vi "Periodic Tasks.vi"(8 "error in":errorcluster) -> ()   [LabVIEW 2012]
doc: "This VI runs in parallel to other tasks. It can contain as many user-defined periodic loops as you need. These can carry out PID or other sorts of timed response."
uses:
  <vilib>/Rock Robotics/SystemInterfaces/Utilities/FPGA_UtilitiesLED Source.ctl
  <vilib>/Rock Robotics/SystemInterfaces/Utilities/FPGA_UtilitiesLED State.ctl
  <vilib>/Rock Robotics/WPI/Solenoid/WPI_SolenoidValue.ctl
  <vilib>/Rock Robotics/WPI/Relay/WPI_RelayValue.ctl
  Robot Global Data.vi
  <vilib>/Rock Robotics/WPI/Solenoid/WPI_SolenoidSetEnum.vi
  <vilib>/Rock Robotics/WPI/Compressor/WPI_CompressorGetSetRefNum.vi
panel:
  out "Pot1 Raw":dbl
  out "Pot1":dbl
  out "PickupError":errorcluster
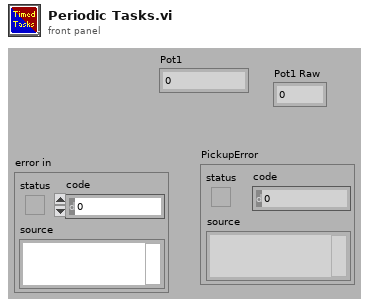
[diagram p1: front panel]
types:
  T1 = typedef "FPGA_UtilitiesLED State.ctl" = enum16{"Off", "On", "Toggle"}
  T2 = typedef "FPGA_UtilitiesLED Source.ctl" = enum16{"User LED", "FPGA LED"}
  T3 = typedef "WPI_SolenoidDevRef.ctl" = cluster{"DevStatus":errorcluster, "Solenoid Module":T4, "Forward Solenoid Channel":T5, "Reverse Solenoid Channel":T5}
  T4 = typedef "FPGA_TypedefSolenoidModule.ctl" = enum16{"Solenoid Module 1", "Solenoid Module 2"}
  T5 = typedef "WPI_SolenoidChannel.ctl" = enum8{"Solenoid 1", "Solenoid 2", "Solenoid 3", "Solenoid 4", "Solenoid 5", "Solenoid 6", "Solenoid 7", "Solenoid 8", "Invalid"}
  T6 = typedef "WPI_RelayDevRef.ctl" = cluster{"DevStatus":errorcluster, "Relay Channel":T7, "Digital Module":T8, "Relay Direction":T9}
  T7 = typedef "FPGA_DIORelayChannel.ctl" = enum8{"Relay 1", "Relay 2", "Relay 3", "Relay 4", "Relay 5", "Relay 6", "Relay 7", "Relay 8", "Invalid"}
  T8 = typedef "FPGA_TypedefDigitalModule.ctl" = enum16{"Digital Module 1", "Digital Module 2"}
  T9 = typedef "WPI_RelayDirection.ctl" = enum16{"Both directions", "Forward only", "Reverse only"}
  T10 = typedef "WPI_MotorControlDeviceRef.ctl" = cluster{"DeviceStatus":errorcluster, "Type":enum16{"PWM", "CAN"}, "PWM":cluster{"Digital Module":T8, "PWM Channel":T11, "DeadBand":T12}, "CAN":cluster{"Device Number":u8, "Control Mode":T13, "Semaphore":T14, "Max Vout":dbl}, "Invert":bool, "TransformRef":T15, "InvTransformRef":T15}
  T11 = typedef "FPGA_DIOPWMChannel.ctl" = enum8{"PWM 1", "PWM 2", "PWM 3", "PWM 4", "PWM 5", "PWM 6", "PWM 7", "PWM 8", "PWM 9", "PWM 10", "Invalid"}
  T12 = typedef "WPI_PWMDeadband.ctl" = cluster{"Name":string, "maxPositivePwm":i32, "minPositivePwm":i32, "centerPwm":i32, "maxNegativePwm":i32, "minNegativePwm":i32, "angularRange":u16}
  T13 = typedef "WPI_CANJaguar_ControlMode.ctl" = enum8{"Percent VBus", "Current", "Speed", "Position", "Voltage"}
  T14 = typedef "Semaphore RefNum" = refnum<k1>
  T15 = typedef "WPI_PWMTransform_ConPane.ctl" = refnum<vi>
  T16 = typedef "WPI_CompressorDevRef.ctl" = cluster{"DevStatus":errorcluster, "DigitalInputDevRef":T17, "RelayDevRef":T6}
  T17 = typedef "WPI_DigitalInputDevRef.ctl" = cluster{"DevStatus":errorcluster, "DIO Channel":T18, "Digital Module":T8}
  T18 = typedef "FPGA_DIOChannel.ctl" = enum8{"DIO 1", "DIO 2", "DIO 3", "DIO 4", "DIO 5", "DIO 6", "DIO 7", "DIO 8", "DIO 9", "DIO 10", "DIO 11", "DIO 12", "DIO 13", "DIO 14", "Invalid"}
  T19 = typedef "WPI_AnalogChannelDevRef.ctl" = cluster{"DevStatus":errorcluster, "Analog Module":T20, "Analog Channel":T21}
  T20 = typedef "FPGA_TypedefAnalogModule.ctl" = enum16{"Analog Module 1", "Analog Module 2"}
  T21 = typedef "FPGA_AIChannel.ctl" = enum8{"AI 1", "AI 2", "AI 3", "AI 4", "AI 5", "AI 6", "AI 7", "AI 8", "Invalid"}
  T22 = enum16{"Reset", "Ready", "Down", "Capture", "Lift", "Swing", "Release"}
  T23 = typedef "WPI_SolenoidValue.ctl" = enum16{"Off", "On", "Forward", "Reverse"}
  T24 = typedef "WPI_RelayValue.ctl" = enum16{"Off", "On", "Forward", "Reverse"}
  T25 = cluster{"PizzaLow":dbl, "PizzaMid":dbl, "PizzaTop":dbl}
  T26 = cluster{"Shoot":bool, "Enable_Targeting":bool, "Shooter":dbl, "LeadScrew":dbl, "Feed":bool, "Pickup":bool, "LiftHooks":bool, "Vision On":bool, "Vision Off":bool, "DownHooks":bool}
  T27 = cluster{"Frisbee_Catch":bool, "Shooter_Ready":bool, "LeadScrewEnd":bool}
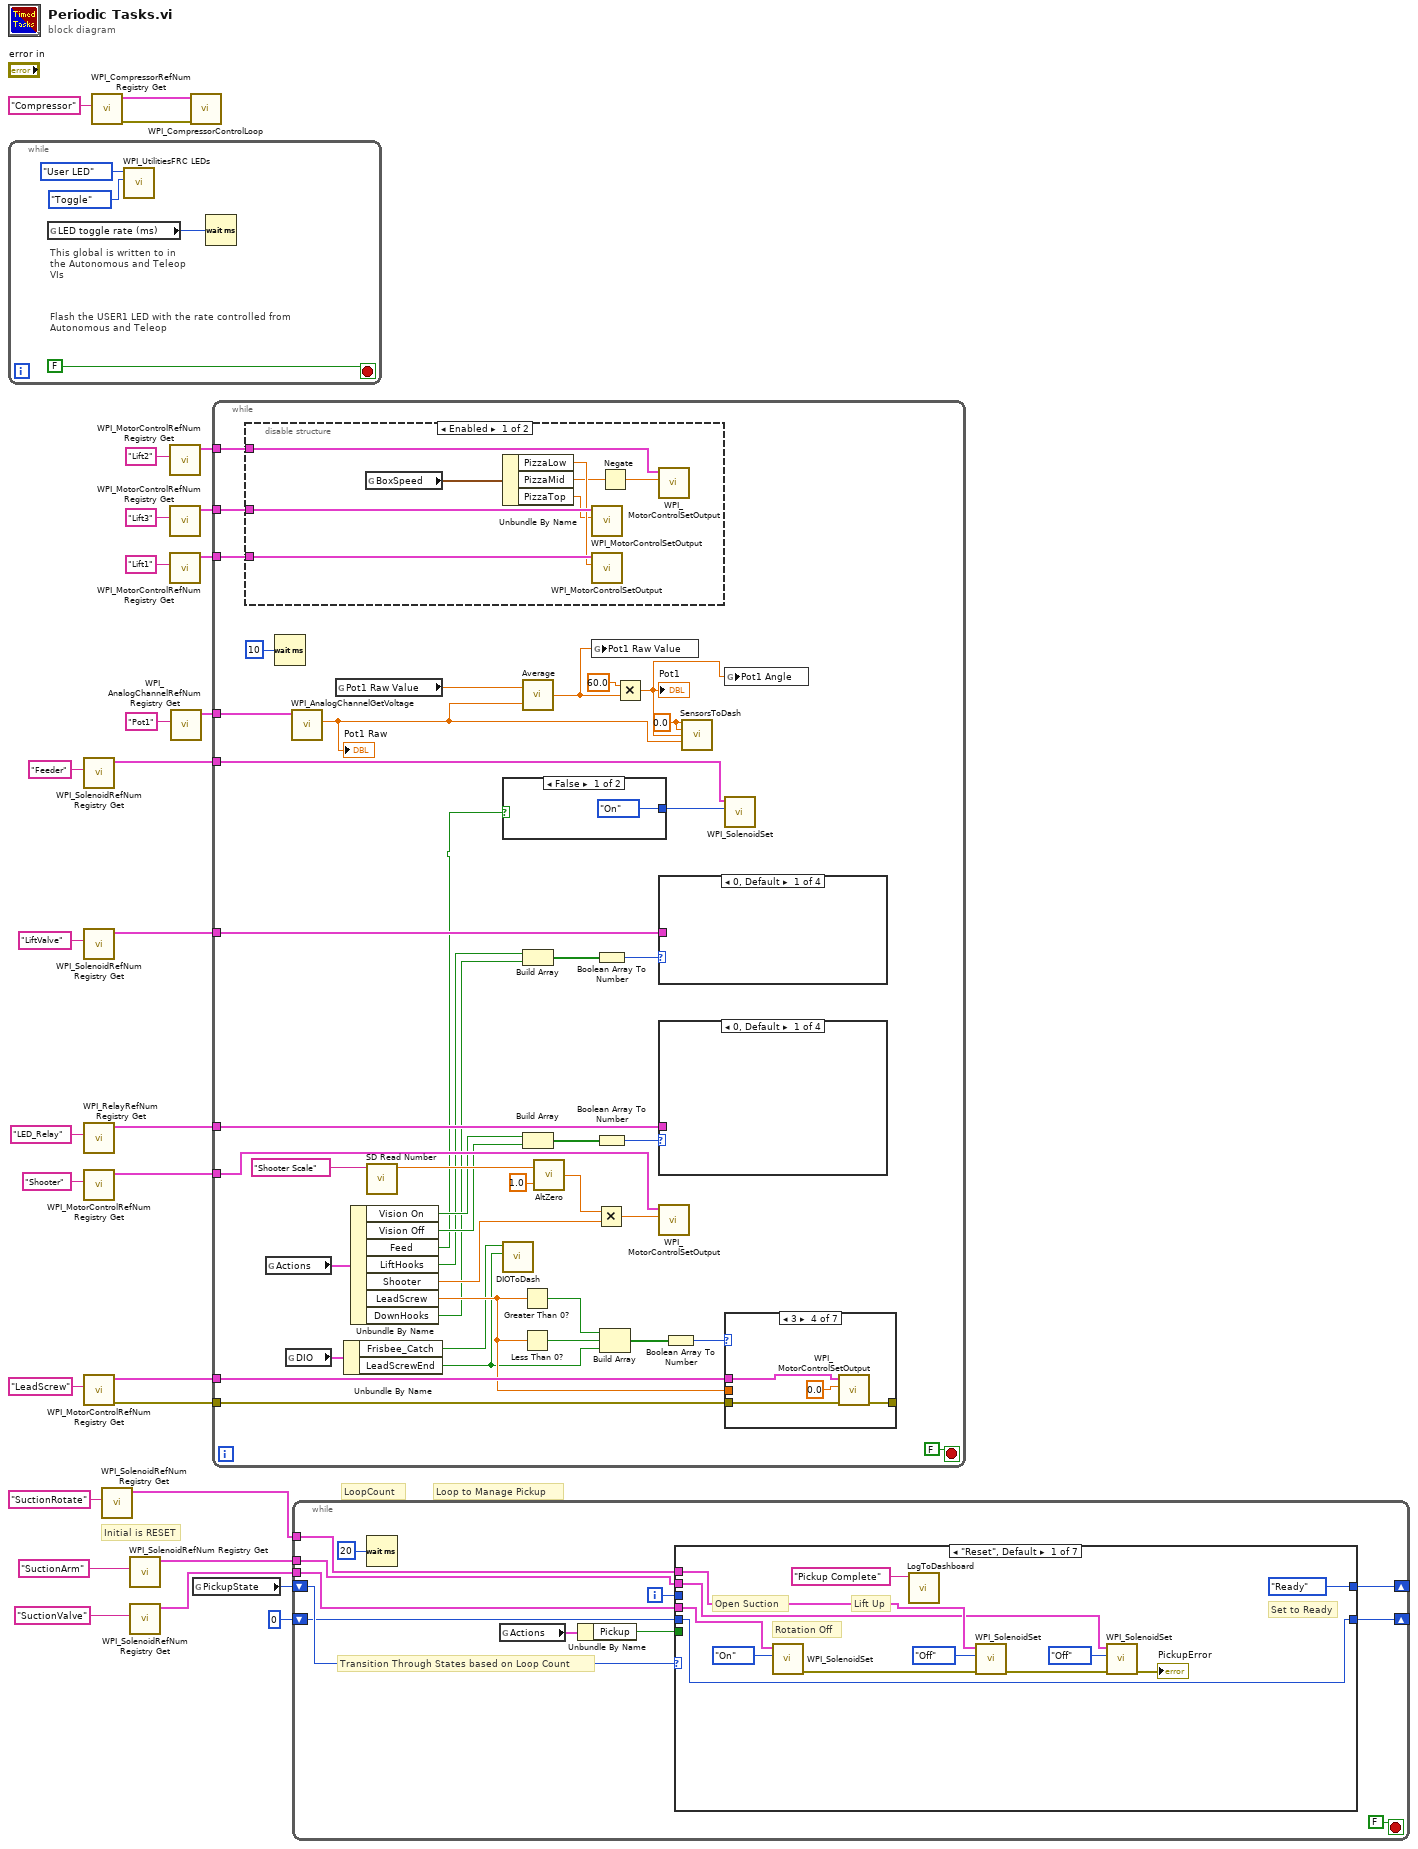
[diagram p0: block diagram]
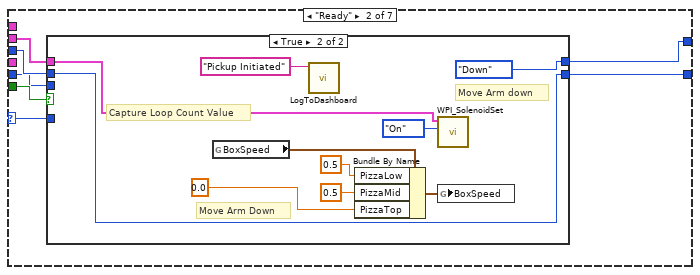
[diagram p2: hidden frame]
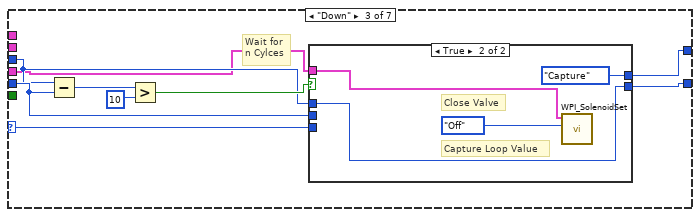
[diagram p4: hidden frame]
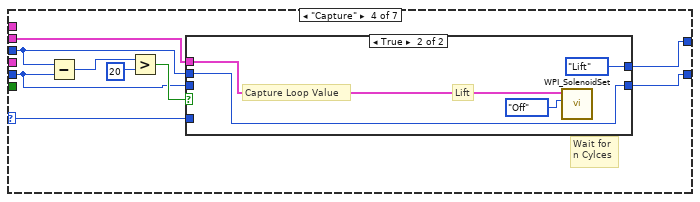
[diagram p6: hidden frame]
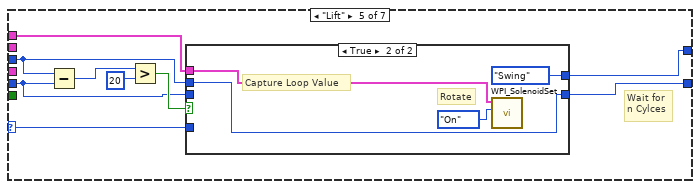
[diagram p8: hidden frame]
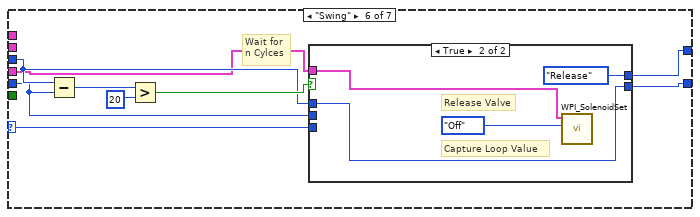
[diagram p10: hidden frame]
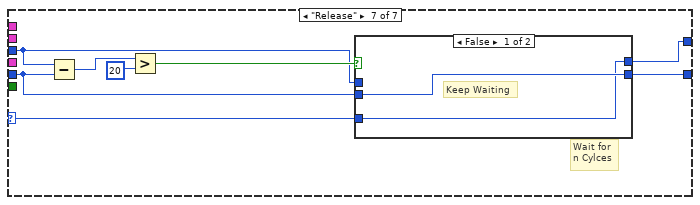
[diagram p12: hidden frame]
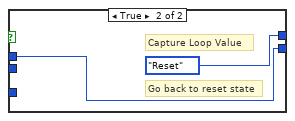
[diagram p13: hidden frame]
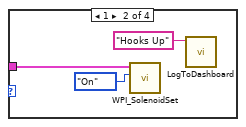
[diagram p14: hidden frame]
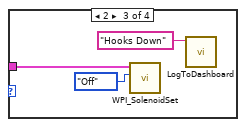
[diagram p15: hidden frame]
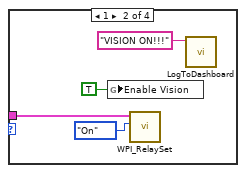
[diagram p18: hidden frame]
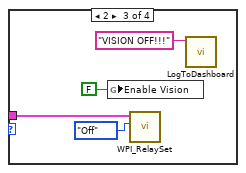
[diagram p19: hidden frame]
diagram:
  # "Initial is RESET"
  # "LoopCount"
  # "Loop to Manage Pickup"
  n1 = while {
    stop <- FALSE stop-if-true
    # "This global is written to in the Autonomous and Teleop VIs"
    # "Flash the USER1 LED with the rate controlled from Autonomous and Teleop"
    n2 = global read "Robot Global Data.vi" "LED toggle rate (ms)"() -> (w31:u32)
    n3 = call <vilib>:"WPI_UtilitiesFRC LEDs.vi"("State"=FPGA_UtilitiesLED_State."Toggle", "LED Type"=FPGA_UtilitiesLED_Source."User LED") -> ()  [unwired: 1 in, 9 out]
    n4 = Wait (ms)(milliseconds to wait=w31) -> ()  [unwired: 1 out]
  }
  n5 = call <vilib>:"WPI_SolenoidRefNum Registry Get.vi"("refnum name"="Feeder") -> ("SolenoidDevRef"=w24:T3)  [unwired: 9 in, 1 out]
  n6 = call <vilib>:"WPI_SolenoidRefNum Registry Get.vi"("refnum name"="LiftValve") -> ("SolenoidDevRef"=w5:T3)  [unwired: 9 in, 1 out]
  n7 = call <vilib>:"WPI_RelayRefNum Registry Get.vi"("refnum name"="LED_Relay") -> ("RelayDevRef"=w3:T6)  [unwired: 9 in, 1 out]
  n8 = call <vilib>:"WPI_MotorControlRefNum Registry Get.vi"("refnum name"="Shooter") -> ("MotorControlDevRef"=w25:T10)  [unwired: 9 in, 1 out]
  n9 = call <vilib>:"WPI_MotorControlRefNum Registry Get.vi"("refnum name"="LeadScrew") -> ("error out"=w2:errorcluster, "MotorControlDevRef"=w27:T10)  [unwired: 9 in]
  n10 = call <vilib>:"WPI_CompressorRefNum Registry Get.vi"("refnum name"="Compressor") -> ("error out"=w29:errorcluster, "CompressorDevRef"=w1:T16)  [unwired: 9 in]
  n11 = call <vilib>:"WPI_SolenoidRefNum Registry Get.vi"("refnum name"="SuctionRotate") -> ("SolenoidDevRef"=w17:T3)  [unwired: 9 in, 1 out]
  n12 = call <vilib>:"WPI_SolenoidRefNum Registry Get.vi"("refnum name"="SuctionArm") -> ("SolenoidDevRef"=w18:T3)  [unwired: 9 in, 1 out]
  n13 = call <vilib>:"WPI_SolenoidRefNum Registry Get.vi"("refnum name"="SuctionValve") -> ("SolenoidDevRef"=w19:T3)  [unwired: 9 in, 1 out]
  n14 = call <vilib>:"WPI_MotorControlRefNum Registry Get.vi"("refnum name"="Lift2") -> ("MotorControlDevRef"=w9:T10)  [unwired: 9 in, 1 out]
  n15 = call <vilib>:"WPI_MotorControlRefNum Registry Get.vi"("refnum name"="Lift3") -> ("MotorControlDevRef"=w10:T10)  [unwired: 9 in, 1 out]
  n16 = call <vilib>:"WPI_MotorControlRefNum Registry Get.vi"("refnum name"="Lift1") -> ("MotorControlDevRef"=w11:T10)  [unwired: 9 in, 1 out]
  n17 = call <vilib>:"WPI_AnalogChannelRefNum Registry Get.vi"("refnum name"="Pot1") -> ("AIDeviceRef"=w7:T19)  [unwired: 9 in, 1 out]
  n18 = call <vilib>:"WPI_CompressorControlLoop.vi"("error in (no error)"=w29, "CompressorDevRef"=w1) -> ()  [unwired: 10 in]
  n19 = global read "Robot Global Data.vi" "PickupState"() -> (w16:T22)
  n20 = while {
    tunnel: w27 -> [w71]
    tunnel: w25 -> [w70]
    tunnel: w24 -> [w68]
    tunnel: w11 -> [w66]
    tunnel: w10 -> [w65]
    tunnel: w9 -> [w64]
    tunnel: w7 -> [w59]
    tunnel: w5 -> [w37]
    tunnel: w3 -> [w44]
    tunnel: w2 -> [w36]
    stop <- FALSE stop-if-true
    w42 = 0.0 ("Gyro1 Angle")
    n21 = disable-structure shown="Enabled" {
      disable-tunnel: w66 -> [w90 _]
      disable-tunnel: w65 -> [w89 _]
      disable-tunnel: w64 -> [w88 _]
      frame Enabled {
        n22 = global read "Robot Global Data.vi" "BoxSpeed"() -> (w91:T25)
        n23 = Unbundle By Name(w91) -> ("PizzaLow"=w87:dbl, "PizzaMid"=w85:dbl, "PizzaTop"=w84:dbl)
        n24 = call <vilib>:"WPI_MotorControlSetOutput.vi"("Output"=w84, "MotorControlDevRef"=w89) -> ()  [unwired: 7 in, 3 out]
        n25 = call <vilib>:"WPI_MotorControlSetOutput.vi"("Output"=w87, "MotorControlDevRef"=w90) -> ()  [unwired: 7 in, 3 out]
        n26 = Negate(x=w85) -> (-x=w86:dbl)
        n27 = call <vilib>:"WPI_MotorControlSetOutput.vi"("Output"=w86, "MotorControlDevRef"=w88) -> ()  [unwired: 7 in, 3 out]
      }
      frame Disabled {
      }
    }
    n28 = global read "Robot Global Data.vi" "Actions"() -> (w69:T26)
    n29 = Wait (ms)(milliseconds to wait=u32 10) -> ()  [unwired: 1 out]
    n30 = global read "Robot Global Data.vi" "DIO"() -> (w54:T27)
    n31 = call <vilib>:"WPI_AnalogChannelGetVoltage.vi"("AIDeviceRef"=w59) -> ("Voltage"=w58:dbl)  [unwired: 8 in, 2 out]
    "Pot1 Raw" <- w58
    n32 = global read "Robot Global Data.vi" "Pot1 Raw Value"() -> (w50:dbl)
    n33 = Unbundle By Name(w54) -> ("Frisbee_Catch"=w53:bool, "LeadScrewEnd"=w52:bool)
    n34 = Unbundle By Name(w69) -> ("Vision On"=w48:bool, "Vision Off"=w47:bool, "Feed"=w35:bool, "LiftHooks"=w41:bool, "Shooter"=w56:dbl, "LeadScrew"=w67:dbl, "DownHooks"=w40:bool)
    n35 = call <vilib>:"SD Read Number.vi"("Name"="Shooter Scale") -> ("Numeric"=w62:dbl)  [unwired: 8 in, 2 out]
    n36 = case shown="False" w35 {
      tunnel: [WPI_SolenoidValue."On" ("Value") WPI_SolenoidValue."Off" ("Value")] -> w51
      frame False {
      }
      frame True {
      }
    }
    n37 = call "DIOToDash.vi"("Lead Screw Max"=w52, "Frisbee Catch"=w53) -> ()  [unwired: 9 in, 1 out]
    n38 = Greater Than 0?(x=w67) -> (x > 0?=w74:bool)
    n39 = Less Than 0?(x=w67) -> (x < 0?=w75:bool)
    n40 = call "Average.vi"("y"=w58, "x"=w50) -> ("(x+y)/2"=w49:dbl)
    n41 = Build Array(w41, w40) -> (w39:bool[])
    n42 = Build Array(w48, w47) -> (w46:bool[])
    n43 = call "AltZero.vi"("z"=1.0, "x"=w62) -> ("y"=w57:dbl)
    n44 = global write "Robot Global Data.vi" "Pot1 Raw Value"(w49) -> ()
    n45 = Multiply(x=w57, y=w56) -> (x*y=w60:dbl)
    n46 = Boolean Array To Number(Boolean array=w39) -> (number=w38:u32)
    n47 = Boolean Array To Number(Boolean array=w46) -> (number=w45:u32)
    n48 = Build Array(w74, w75, w52) -> (w73:bool[])
    n49 = Multiply(x=60.0, y=w49) -> (x*y=w43:dbl)
    "Pot1" <- w43
    n50 = case shown="0, Default" w38 {
      tunnel: w37 -> [_ w79 w82 _]
      frame 0, Default {
      }
      frame 1 {
        n51 = call-poly <vilib>:"WPI_SolenoidSet.vi"("Value"=WPI_SolenoidValue."On", "SolenoidDevRef"=w79) -> ()  [unwired: 8 in, 2 out]
        n52 = call "LogToDashboard.vi"("Info"="Hooks Up") -> ()  [unwired: 10 in, 1 out]
      }
      frame 2 {
        n53 = call-poly <vilib>:"WPI_SolenoidSet.vi"("Value"=WPI_SolenoidValue."Off", "SolenoidDevRef"=w82) -> ()  [unwired: 8 in, 2 out]
        n54 = call "LogToDashboard.vi"("Info"="Hooks Down") -> ()  [unwired: 10 in, 1 out]
      }
      frame 3 {
      }
    }
    n55 = case shown="0, Default" w45 {
      tunnel: w44 -> [_ w94 w97 _]
      frame 0, Default {
      }
      frame 1 {
        n56 = global write "Robot Global Data.vi" "Enable Vision"(TRUE) -> ()
        n57 = call <vilib>:"WPI_RelaySet.vi"("RelayValue"=WPI_RelayValue."On", "RelayDevRef"=w94) -> ()  [unwired: 8 in, 2 out]
        n58 = call "LogToDashboard.vi"("Info"="VISION ON!!!") -> ()  [unwired: 10 in, 1 out]
      }
      frame 2 {
        n59 = global write "Robot Global Data.vi" "Enable Vision"(FALSE) -> ()
        n60 = call <vilib>:"WPI_RelaySet.vi"("RelayValue"=WPI_RelayValue."Off", "RelayDevRef"=w97) -> ()  [unwired: 8 in, 2 out]
        n61 = call "LogToDashboard.vi"("Info"="VISION OFF!!!") -> ()  [unwired: 10 in, 1 out]
      }
      frame 3 {
      }
    }
    n62 = call <vilib>:"WPI_MotorControlSetOutput.vi"("Output"=w60, "MotorControlDevRef"=w70) -> ()  [unwired: 7 in, 3 out]
    n63 = Boolean Array To Number(Boolean array=w73) -> (number=w72:u32)
    n64 = call "SensorsToDash.vi"("Gyro1 Angle"=w42, "Gyro1Raw"=w42, "Pot1 Angle"=w43, "Pot1Raw"=w58) -> ()  [unwired: 11 in, 1 out]
    n65 = global write "Robot Global Data.vi" "Pot1 Angle"(w43) -> ()
    n66 = call-poly <vilib>:"WPI_SolenoidSet.vi"("Value"=w51, "SolenoidDevRef"=w68) -> ()  [unwired: 8 in, 2 out]
    n67 = case shown="3" w72 {
      tunnel: w67 -> [_ w109 w113 _ _ _ w128]
      tunnel: w71 -> [w104 w108 w112 w117 w121 w125 w129]
      tunnel: w36 -> [w103 w106 w111 w115 w118 w122 w126]
      tunnel: [w102 w107 w110 w114 w119 w123 w127] -> _
      frame 0, Default {
        n68 = call <vilib>:"WPI_MotorControlSetOutput.vi"("error in (no error)"=w103, "Output"=0.0, "MotorControlDevRef"=w104) -> ("error out"=w102:errorcluster)  [unwired: 6 in, 2 out]
      }
      frame 1 {
        n69 = call <vilib>:"WPI_MotorControlSetOutput.vi"("error in (no error)"=w106, "Output"=w109, "MotorControlDevRef"=w108) -> ("error out"=w107:errorcluster)  [unwired: 6 in, 2 out]
      }
      frame 2 {
        n70 = call <vilib>:"WPI_MotorControlSetOutput.vi"("error in (no error)"=w111, "Output"=w113, "MotorControlDevRef"=w112) -> ("error out"=w110:errorcluster)  [unwired: 6 in, 2 out]
      }
      frame 3 {
        n71 = call <vilib>:"WPI_MotorControlSetOutput.vi"("error in (no error)"=w115, "Output"=0.0, "MotorControlDevRef"=w117) -> ("error out"=w114:errorcluster)  [unwired: 6 in, 2 out]
      }
      frame 4 {
        n72 = call <vilib>:"WPI_MotorControlSetOutput.vi"("error in (no error)"=w118, "Output"=0.0, "MotorControlDevRef"=w121) -> ("error out"=w119:errorcluster)  [unwired: 6 in, 2 out]
      }
      frame 5 {
        n73 = call <vilib>:"WPI_MotorControlSetOutput.vi"("error in (no error)"=w122, "Output"=0.0, "MotorControlDevRef"=w125) -> ("error out"=w123:errorcluster)  [unwired: 6 in, 2 out]
      }
      frame 6 {
        n74 = call <vilib>:"WPI_MotorControlSetOutput.vi"("error in (no error)"=w126, "Output"=w128, "MotorControlDevRef"=w129) -> ("error out"=w127:errorcluster)  [unwired: 6 in, 2 out]
      }
    }
  }
  n75 = while {
    tunnel: w19 -> [w139]
    tunnel: w18 -> [w138]
    tunnel: w17 -> [w137]
    shift-right: [w136] -> _
    shift-left: w16 -> [w135]
    shift-right: [w130] -> _
    shift-left: 0 -> [w131]
    i -> [w132]
    stop <- FALSE stop-if-true
    # "Transition Through States based on Loop Count"
    n76 = Wait (ms)(milliseconds to wait=u32 20) -> ()  [unwired: 1 out]
    n77 = global read "Robot Global Data.vi" "Actions"() -> (w134:T26)
    n78 = Unbundle By Name(w134) -> ("Pickup"=w133:bool)
    n79 = case shown="\"Reset\", Default" w135 {
      selector: w135 -> [_ w154 w176 w193 w204 w219 w235]
      tunnel: w139 -> [w153 _ w173 _ _ w218 _]
      tunnel: w138 -> [w145 w158 _ w190 _ _ _]
      tunnel: w137 -> [w146 _ _ _ w203 _ _]
      tunnel: [T22."Ready" ("PickupState") w159 w175 w189 w205 w223 w234] -> w136
      tunnel: w133 -> [_ w160 _ _ _ _ _]
      tunnel: w132 -> [_ w157 w174 w192 w208 w221 w237]
      tunnel: w131 -> [w147 w155 w178 w191 w207 w220 w236]
      tunnel: [w147 w156 w177 w188 w206 w222 w233] -> w130
      frame "Reset", Default {
        # "Set to Ready"
        # "Rotation Off"
        # "Lift Up"
        # "Open Suction"
        n80 = call-poly <vilib>:"WPI_SolenoidSet.vi"("Value"=WPI_SolenoidValue."On", "SolenoidDevRef"=w153) -> ("error out"=w150:errorcluster)  [unwired: 8 in, 1 out]
        n81 = call "LogToDashboard.vi"("Info"="Pickup Complete") -> ()  [unwired: 10 in, 1 out]
        n82 = call-poly <vilib>:"WPI_SolenoidSet.vi"("error in (no error)"=w150, "Value"=WPI_SolenoidValue."Off", "SolenoidDevRef"=w146) -> ("error out"=w144:errorcluster)  [unwired: 7 in, 1 out]
        n83 = call-poly <vilib>:"WPI_SolenoidSet.vi"("error in (no error)"=w144, "Value"=WPI_SolenoidValue."Off", "SolenoidDevRef"=w145) -> ("error out"=→"PickupError":errorcluster)  [unwired: 7 in, 1 out]
      }
      frame "Ready" {
        n84 = case shown="True" w160 {
          tunnel: [w161 T22."Down" ("PickupState")] -> w159
          tunnel: w158 -> [_ w171]
          tunnel: w157 -> [_ w169]
          tunnel: [w162 w169] -> w156
          tunnel: w155 -> [w162 _]
          tunnel: w154 -> [w161 _]
          frame False {
            # "Pass state\nand Loop\nCount"
          }
          frame True {
            # "Move Arm down"
            # "Capture Loop Count Value"
            # "Move Arm Down"
            n85 = global read "Robot Global Data.vi" "BoxSpeed"() -> (w168:T25)
            n86 = call "LogToDashboard.vi"("Info"="Pickup Initiated") -> ()  [unwired: 10 in, 1 out]
            n87 = Bundle By Name(cluster=w168, "PizzaLow"=0.5, "PizzaMid"=0.5, "PizzaTop"=0.0) -> (w164:T25)
            n88 = call-poly <vilib>:"WPI_SolenoidSet.vi"("Value"=WPI_SolenoidValue."On", "SolenoidDevRef"=w171) -> ()  [unwired: 8 in, 2 out]
            n89 = global write "Robot Global Data.vi" "BoxSpeed"(w164) -> ()
          }
        }
      }
      frame "Down" {
        # "Wait for\nn Cylces"
        n90 = Subtract(x=w174, y=w178) -> (x-y=w181:i32)
        n91 = Greater?(x=w181, y=10) -> (0:w179:bool)
        n92 = case shown="True" w179 {
          tunnel: w178 -> [w183 _]
          tunnel: [w183 w187] -> w177
          tunnel: w176 -> [w182 _]
          tunnel: [w182 T22."Capture" ("PickupState")] -> w175
          tunnel: w174 -> [_ w187]
          tunnel: w173 -> [_ w186]
          frame False {
            # "Keep Waiting"
          }
          frame True {
            # "Capture Loop Value"
            # "Close Valve"
            n93 = call-poly <vilib>:"WPI_SolenoidSet.vi"("Value"=WPI_SolenoidValue."Off", "SolenoidDevRef"=w186) -> ()  [unwired: 8 in, 2 out]
          }
        }
      }
      frame "Capture" {
        # "Wait for\nn Cylces"
        n94 = Subtract(x=w192, y=w191) -> (x-y=w196:i32)
        n95 = Greater?(x=w196, y=20) -> (0:w194:bool)
        n96 = case shown="True" w194 {
          tunnel: w191 -> [w198 _]
          tunnel: [w198 w202] -> w188
          tunnel: w193 -> [w197 _]
          tunnel: [w197 T22."Lift" ("PickupState")] -> w189
          tunnel: w192 -> [_ w202]
          tunnel: w190 -> [_ w201]
          frame False {
            # "Keep Waiting"
          }
          frame True {
            # "Capture Loop Value"
            # "Lift"
            n97 = call-poly <vilib>:"WPI_SolenoidSet.vi"("Value"=WPI_SolenoidValue."Off", "SolenoidDevRef"=w201) -> ()  [unwired: 8 in, 2 out]
          }
        }
      }
      frame "Lift" {
        # "Wait for\nn Cylces"
        n98 = Subtract(x=w208, y=w207) -> (x-y=w211:i32)
        n99 = Greater?(x=w211, y=20) -> (0:w209:bool)
        n100 = case shown="True" w209 {
          tunnel: w207 -> [w213 _]
          tunnel: [w213 w217] -> w206
          tunnel: w204 -> [w212 _]
          tunnel: [w212 T22."Swing" ("PickupState")] -> w205
          tunnel: w208 -> [_ w217]
          tunnel: w203 -> [_ w216]
          frame False {
            # "Keep Waiting"
          }
          frame True {
            # "Capture Loop Value"
            # "Rotate"
            n101 = call-poly <vilib>:"WPI_SolenoidSet.vi"("Value"=WPI_SolenoidValue."On", "SolenoidDevRef"=w216) -> ()  [unwired: 8 in, 2 out]
          }
        }
      }
      frame "Swing" {
        # "Wait for\nn Cylces"
        n102 = Subtract(x=w221, y=w220) -> (x-y=w226:i32)
        n103 = Greater?(x=w226, y=20) -> (0:w224:bool)
        n104 = case shown="True" w224 {
          tunnel: w220 -> [w228 _]
          tunnel: [w228 w232] -> w222
          tunnel: w219 -> [w227 _]
          tunnel: [w227 T22."Release" ("PickupState")] -> w223
          tunnel: w221 -> [_ w232]
          tunnel: w218 -> [_ w231]
          frame False {
            # "Keep Waiting"
          }
          frame True {
            # "Capture Loop Value"
            # "Release Valve"
            n105 = call-poly <vilib>:"WPI_SolenoidSet.vi"("Value"=WPI_SolenoidValue."Off", "SolenoidDevRef"=w231) -> ()  [unwired: 8 in, 2 out]
          }
        }
      }
      frame "Release" {
        # "Wait for\nn Cylces"
        n106 = Subtract(x=w237, y=w236) -> (x-y=w240:i32)
        n107 = Greater?(x=w240, y=20) -> (0:w238:bool)
        n108 = case shown="False" w238 {
          tunnel: w236 -> [w242 _]
          tunnel: [w242 w244] -> w233
          tunnel: w235 -> [w241 _]
          tunnel: [w241 T22."Reset" ("PickupState")] -> w234
          tunnel: w237 -> [_ w244]
          frame False {
            # "Keep Waiting"
          }
          frame True {
            # "Go back to reset state"
            # "Capture Loop Value"
          }
        }
      }
    }
  }
